vi "Read Caller.vi"(8 "error in (no error)":errorcluster, 11 "RQMHStartup in":refnum<class "RQMHStartup.lvclass">) -> (0 "error out":errorcluster, 2 "Caller":string, 3 "RQMHStartup out":refnum<class "RQMHStartup.lvclass">)   [LabVIEW 2024, in "RQMHStartup.lvclass"]
uses:
  RQMHStartup.lvclass
  RQMHStartup.lvclass/RQMHStartup.ctl
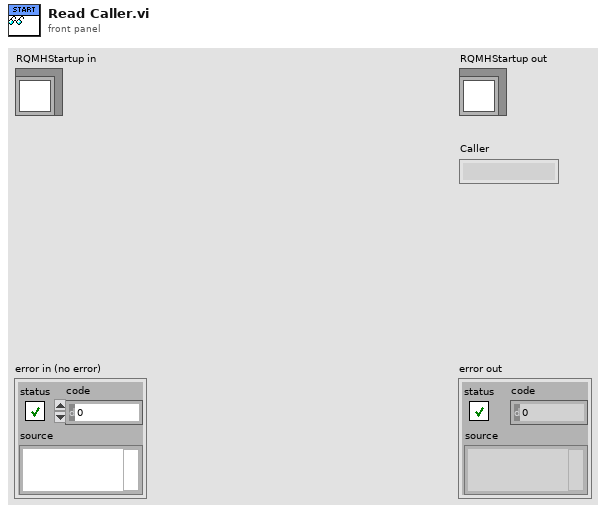
[diagram p1: front panel]
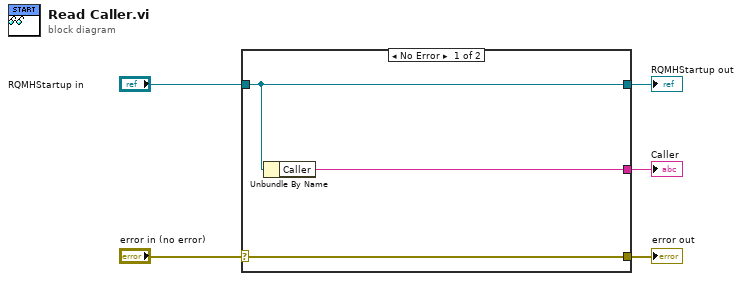
[diagram p0: block diagram]
diagram:
  n1 = case shown="No Error" "error in (no error)" {
    selector: "error in (no error)" -> [w8 w9]
    tunnel: [w8 w9] -> w4
    tunnel: [w7 w10] -> w2
    tunnel: "RQMHStartup in" -> [w7 w10]
    tunnel: [w6 _] -> w1
    frame No Error {
      n2 = Unbundle By Name(w7) -> ("Caller"=w6:string)
    }
    frame Error {
    }
  }
  "error out" <- w4
  "RQMHStartup out" <- w2
  "Caller" <- w1
